vi "publish_builder.vi"(11 "topic":string="/chatter") -> (3 "?":cluster{"op":string, "topic":string})   [LabVIEW 2014]
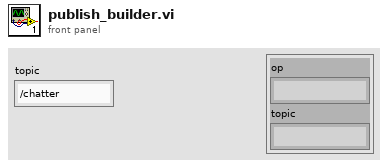
[diagram p1: front panel]
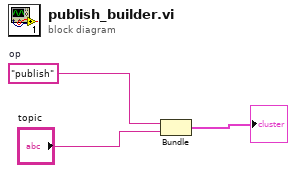
[diagram p0: block diagram]
diagram:
  w3 = "publish"  # op
  n1 = Bundle("op"=w3, "topic"="topic") -> (→"?":cluster{"op":string, "topic":string})  [unwired: 1 in]
